vi "packAFrameFromData.vi"(1 "src data":u8[](array[numeric])) -> (0 "dst frame":u8[](array[numeric]))   [LabVIEW 2014]
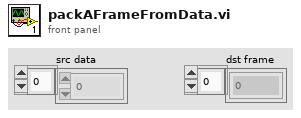
[diagram p1: front panel]
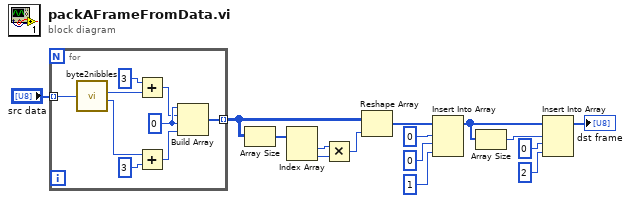
[diagram p0: block diagram]
diagram:
  n1 = for {
    tunnel: "src data" -> [w24] mode=indexing
    tunnel: [w20] -> w1 mode=indexing
    w21 = u8 0 ("element")
    n2 = call "byte2nibbles.vi"("byte"=w24) -> ("high nibble"=w23:u8, "low nibble"=w22:u8)  [unwired: 2 in]
    n3 = Add(x=u8 3, y=w23) -> (x+y=w19:u8)
    n4 = Add(x=w22, y=u8 3) -> (x+y=w18:u8)
    n5 = Build Array(w21, w19, w21, w18) -> (w20:u8[])
  }
  n6 = Array Size(array=w1) -> (size(s)=w2:i32[])
  n7 = Index Array(array=w2) -> (element #1=w4:i32, element #2=w3:i32)  [unwired: 2 in]
  n8 = Multiply(x=w4, y=w3) -> (x*y=w5:i32)
  n9 = Reshape Array(w1, w5) -> (w11:u8[])
  n10 = Insert Into Array(array=w11, index=0, new element #1=u8 0 ("new element/subarray"), new element #2=u8 1 ("new element/subarray")) -> (w9:u8[])
  n11 = Array Size(array=w9) -> (size(s)=w10:i32)
  n12 = Insert Into Array(array=w9, index=w10, new element #1=u8 0 ("new element/subarray"), new element #2=u8 2 ("new element/subarray")) -> (→"dst frame":u8[])
